vi "Status Updater Manual Test.vi"() -> ()   [LabVIEW 2014]
uses:
  Core/Shared/Classes/Status Updater/Status Updater.lvclass/Status Updater.ctl
  Core/Shared/Classes/Status Updater/Status Updater.lvclass
  Core/Shared/Classes/Status Events/Status Events.lvclass
panel:
  in  "stop":bool
  out "Numeric 2":dbl
  out "String":string
  in  "Numeric":dbl
  in  "Text":string
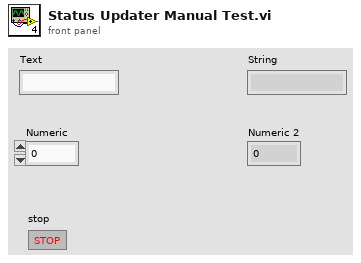
[diagram p1: front panel]
types:
  T1 = cluster{"Event Registration Refnum":refnum<event-registration>, "Event Registration Refnum":refnum<event-registration>}
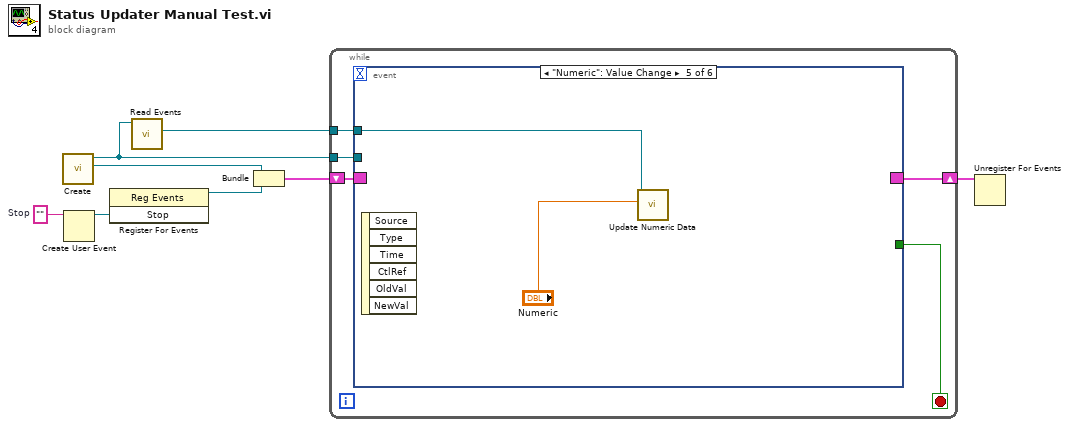
[diagram p0: block diagram]
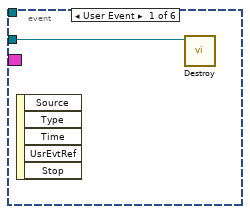
[diagram p2: hidden frame]
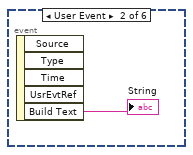
[diagram p3: hidden frame]
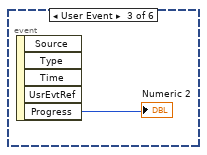
[diagram p4: hidden frame]
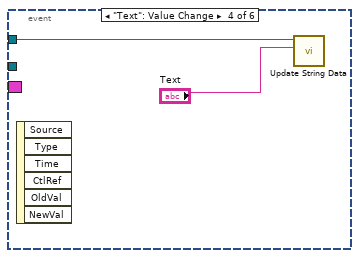
[diagram p5: hidden frame]
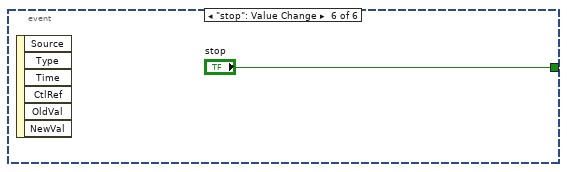
[diagram p6: hidden frame]
diagram:
  w8 = ""  # Stop
  n1 = call "Create.vi"() -> ("Event Registration Refnum"=w6:refnum<event-registration>, "Status Updater out"=w2:refnum<class "Status Updater.lvclass">)  [unwired: 9 in, 1 out]
  n2 = Create User Event(user event datatype=w8) -> (user event=w7:refnum<user-event>)  [unwired: 1 in, 1 out]
  n3 = register-events(w7) -> (reference out=w5:refnum<event-registration>)  [unwired: 2 in, 1 out]
  n4 = call "Read Events.vi"("Status Updater in"=w2) -> ("Status Events"=w1:refnum<class "Status Events.lvclass">)  [unwired: 10 in]
  n5 = Bundle("Event Registration Refnum"=w6, "Event Registration Refnum"=w5) -> (w4:T1)  [unwired: 1 in]
  n6 = while {
    tunnel: w2 -> [w11]
    shift-right: [w12] -> w3
    shift-left: w4 -> [w13]
    tunnel: w1 -> [w9]
    stop <- w10 stop-if-true
    n7 = event shown="[4] \"Numeric\": Value Change" {
      selector: w13 -> [_ _ _ _ _ _]
      dyn-events: [_ _ _ _ _ _] -> w12
      timeout: _ -> [_ _ _ _ _ _]
      tunnel: w11 -> [w14 _ _ _ _ _]
      tunnel: [_ _ _ _ _ "stop"] -> w10
      tunnel: w9 -> [_ _ _ w17 w20 _]
      event User Event {
        n8 = event-data() -> ()  [unwired: 1 in, 5 out]
        n9 = call "Destroy.vi"("Status Updater in"=w14) -> ()  [unwired: 10 in, 1 out]
      }
      event User Event {
        n10 = event-data() -> ("Build Text"=→"String":string)  [unwired: 1 in, 4 out]
      }
      event User Event {
        n11 = event-data() -> ("Progress"=→"Numeric 2":u32)  [unwired: 1 in, 4 out]
      }
      event "Text": Value Change {
        n12 = event-data() -> ()  [unwired: 1 in, 6 out]
        n13 = call "Update String Data.vi"("String Data"="Text", "Status Updater in"=w17) -> ()  [unwired: 8 in, 2 out]
      }
      event "Numeric": Value Change {
        n14 = event-data() -> ()  [unwired: 1 in, 6 out]
        n15 = call "Update Numeric Data.vi"("Numeric Data"="Numeric", "Status Updater in"=w20) -> ()  [unwired: 8 in, 2 out]
      }
      event "stop": Value Change {
        n16 = event-data() -> ()  [unwired: 1 in, 6 out]
      }
    }
  }
  n17 = Unregister For Events(event registration refnum=w3) -> ()  [unwired: 1 in, 1 out]
